vi "CRYHarmonics array to list.vi"(10 "Harmonics array":string[](array[string]), 11 "Items":string[](array[string])) -> (1 "Checkoffs out":bool[](array[boolean]), 2 "Symbols out":i32[](array[numeric]), 3 "Items out":string[](array[string]))   [LabVIEW 2013]
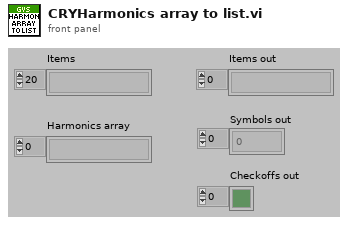
[diagram p1: front panel]
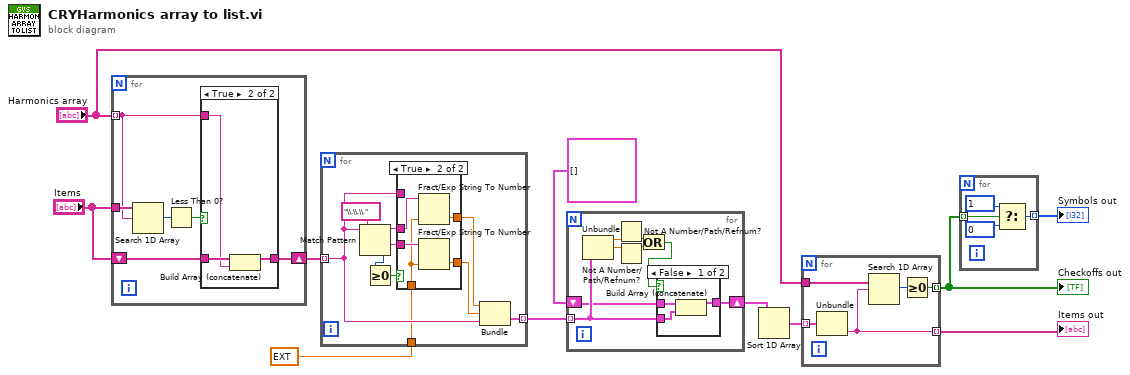
[diagram p0: block diagram]
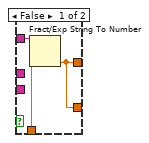
[diagram p3: hidden frame]
diagram:
  n1 = for {
    shift-right: [w12] -> w9
    shift-left: "Items" -> [w14]
    tunnel: "Harmonics array" -> [w13] mode=indexing
    tunnel: "Items" -> [w17]
    n2 = Search 1D Array(1D array=w17, element=w13) -> (index of element=w16:i32)  [unwired: 1 out]
    n3 = Less Than 0?(x=w16) -> (x < 0?=w15:bool)
    n4 = case shown="True" w15 {
      tunnel: w14 -> [w18 w21]
      tunnel: w13 -> [_ w20]
      tunnel: [w18 w19] -> w12
      frame False {
      }
      frame True {
        n5 = Build Array (concatenate)(w21, w20) -> (w19:string[])
      }
    }
  }
  n6 = for {
    tunnel: w9 -> [w28] mode=indexing
    tunnel: [w27] -> w3 mode=indexing
    tunnel: ext nan ("default (0 dbl)") -> [w22]
    n7 = Match Pattern(string=w28, regular expression="\\.\\.\\.") -> (before substring=w26:string, after substring=w25:string, offset past match=w31:i32)  [unwired: 2 out]
    n8 = Greater Or Equal To 0?(x=w31) -> (x >= 0?=w30:bool)
    n9 = case shown="True" w30 {
      tunnel: w28 -> [w34 _]
      tunnel: [w33 w38] -> w23
      tunnel: w26 -> [_ w39]
      tunnel: w25 -> [_ w37]
      tunnel: [w33 w36] -> w24
      tunnel: w22 -> [w32 w35]
      frame False {
        n10 = Fract/Exp String To Number(string=w34, default (0 dbl)=w32) -> (number=w33:ext)  [unwired: 3 out]
      }
      frame True {
        n11 = Fract/Exp String To Number(string=w39, default (0 dbl)=w35) -> (number=w38:ext)  [unwired: 3 out]
        n12 = Fract/Exp String To Number(string=w37, default (0 dbl)=w35) -> (number=w36:ext)  [unwired: 3 out]
      }
    }
    n13 = Bundle(w23, w24, "String"=w28) -> (w27:cluster{ext, ext, "String":string})  [unwired: 1 out]
  }
  n14 = for {
    shift-right: [w46] -> w2
    shift-left: cluster{ext, ext, "String":string}[] [] -> [w44]
    tunnel: w3 -> [w45] mode=indexing
    n15 = Unbundle(w45) -> (w47:ext, w43:ext)  [unwired: 1 out]
    n16 = Not A Number/Path/Refnum?(number/path/refnum=w47) -> (NaN/Path/Refnum?=w42:bool)
    n17 = Not A Number/Path/Refnum?(number/path/refnum=w43) -> (NaN/Path/Refnum?=w41:bool)
    n18 = Or(x=w42, y=w41) -> (x .or. y?=w40:bool)
    n19 = case shown="False" w40 {
      tunnel: w45 -> [w48 _]
      tunnel: [w50 w51] -> w46
      tunnel: w44 -> [w49 w51]
      frame False {
        n20 = Build Array (concatenate)(w49, w48) -> (w50:cluster{ext, ext, "String":string}[])
      }
      frame True {
      }
    }
  }
  n21 = Sort 1D Array(array=w2) -> (sorted array=w10:cluster{ext, ext, "String":string}[])
  n22 = for {
    tunnel: w10 -> [w56] mode=indexing
    tunnel: [w55] -> w5 mode=indexing
    tunnel: "Harmonics array" -> [w54]
    tunnel: [w52] -> w6 mode=indexing
    n23 = Unbundle(w56) -> ("String"=w55:string)  [unwired: 2 out]
    n24 = Search 1D Array(1D array=w54, element=w55) -> (index of element=w53:i32)  [unwired: 1 out]
    n25 = Greater Or Equal To 0?(x=w53) -> (x >= 0?=w52:bool)
  }
  "Checkoffs out" <- w6
  "Items out" <- w5
  n26 = for {
    tunnel: w6 -> [w60] mode=indexing
    tunnel: [w59] -> w7 mode=indexing
    n27 = Select(t=1, s=w60, f=0) -> (s? t:f=w59:i32)
  }
  "Symbols out" <- w7
